vi "Write Measured.vi"(8 "error in":errorcluster, 10 "Measured":waveform(dbl)[](array[waveform]), 11 "Instruments in":refnum<class "Instruments.lvclass">) -> (0 "error out":errorcluster, 3 "Instruments out":refnum<class "Instruments.lvclass">)   [LabVIEW 2023, in "Instruments.lvlib" / "Instruments.lvclass"]
uses:
  Library/Instruments.lvclass
  Library/Instruments.lvclass/Instruments.ctl
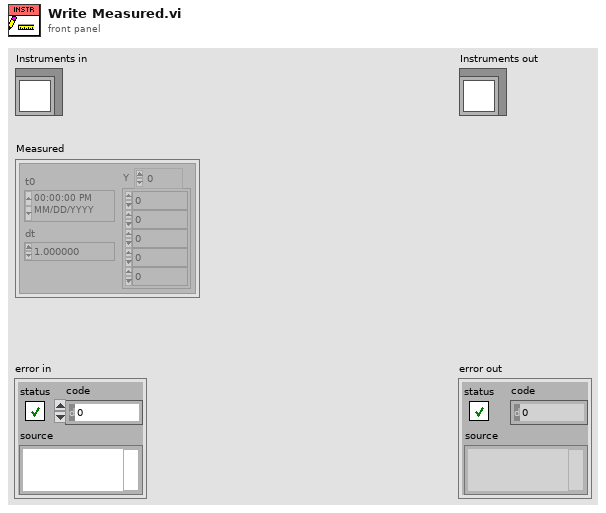
[diagram p1: front panel]
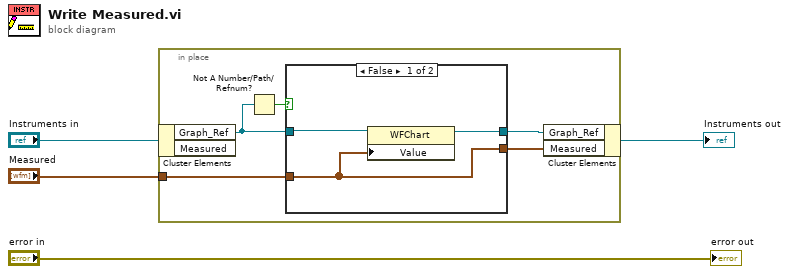
[diagram p0: block diagram]
diagram:
  n1 = in-place {
    in-place-border: "Measured" -> [w6]
    n2 = in-place-cluster #1("Instruments in") -> ("Graph_Ref"=w7:refnum<vi>)  [unwired: 1 out]
    n3 = Not A Number/Path/Refnum?(number/path/refnum=w7) -> (NaN/Path/Refnum?=w9:bool)
    n4 = case shown="False" w9 {
      tunnel: [w11 w14] -> w8
      tunnel: w7 -> [w12 w14]
      tunnel: w6 -> [w10 w13]
      tunnel: [w10 w13] -> w5
      frame False {
        n5 = property class="WFChart"(reference=w12, "Value"=w10) -> (reference out=w11:refnum<vi>)  [unwired: 1 in, 1 out]
      }
      frame True {
      }
    }
    n6 = in-place-cluster #1("Graph_Ref"=w8, "Measured"=w5) -> (→"Instruments out":refnum<class "Instruments.lvclass">)
  }
  "error out" <- "error in"
